vi "audio-stim2.vi"(11 "Stimulus List":dbl[][](array[numeric])) -> (3 "Playing":bool caption="Playing stimulus")   [LabVIEW 2009]
uses:
  <vilib>/DAQmx/create/channels.llb/DAQmx Create Channel (DO-Digital Output).vi
  <vilib>/DAQmx/write.llb/DAQmx Write (Digital U16 1Chan 1Samp).vi
  <vilib>/DAQmx/create/channels.llb/DAQmx Create Channel (AO-Voltage-Basic).vi
  <vilib>/DAQmx/configure/timing.llb/DAQmx Timing (Use Waveform).vi
  <vilib>/DAQmx/write.llb/DAQmx Write (Analog Wfm 1Chan NSamp).vi
panel:
  in  "Total Trials":i32 min=1 step=1
  out "Total Played":i32 caption="Total Played or Cued"
  in  "Save Stimulus List":bool
  in  "Load Stimulus List":bool
  out "Stimulus List Path":path
  out "Log File Path":path
  in  "Play Interval Jitter (s)":dbl
  in  "Play Interval (s)":dbl
  out "error out":errorcluster
  in  "DO Ports":tag caption="DO Ports\n(\"browse\" and select two 8 bit ports)"
  in  "Sound AO Channel":tag
  out "Curr Param":dbl[](array[numeric]) caption="Current (or Cued) Trial Parameters"
  in  "Sampling Rate":dbl
  in  "stop":bool
  in  "Play":bool
  out "Current (or Cued) Waveform":waveform(dbl)(graph)
  out "Waiting":bool
  # "Stim#, Stim Type, Duration, Amplitude, Param 1, Param 2, Param 3, Param 4"
  # "Stim Type 1 DC (no parameters, just amplitude)"
  # "Stim Type 3 Pure Tone (param1 = frequency)"
  # "Stim Type 4 FM Sweep (param1 = start frequency, param2 = end frequency)"
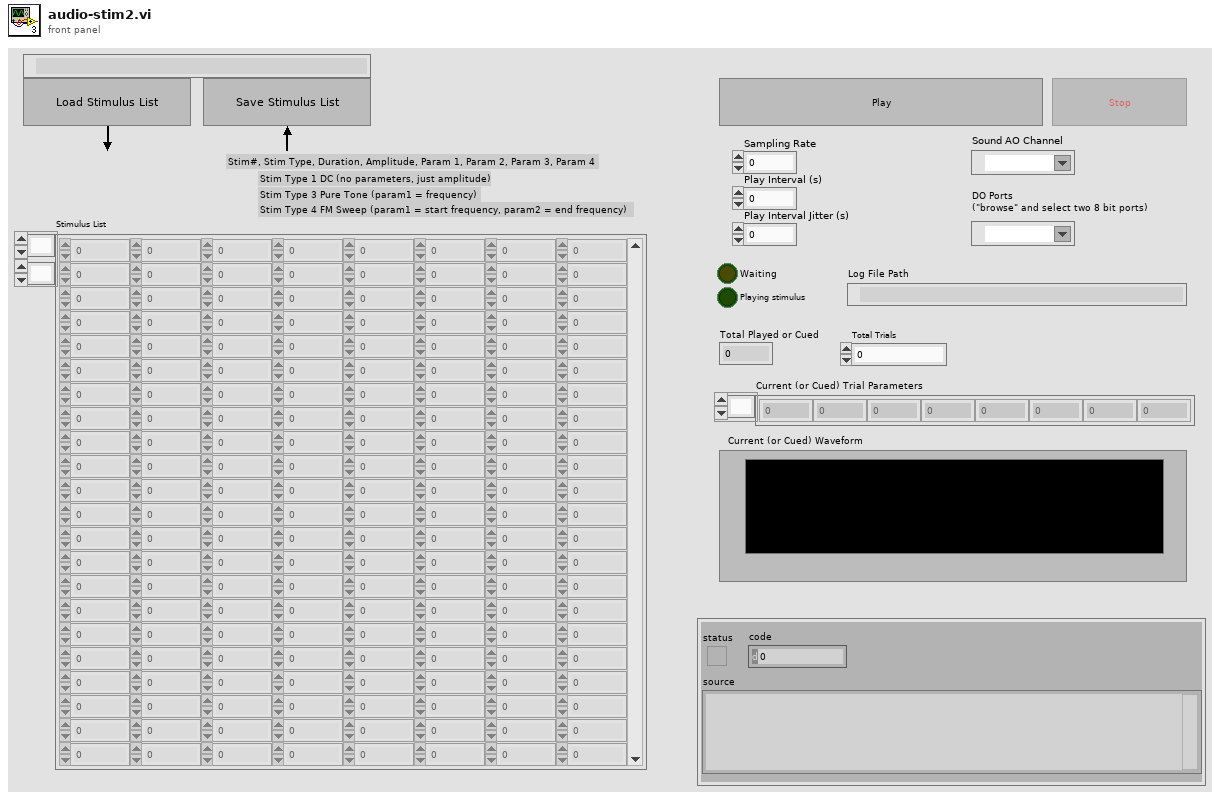
[diagram p1: front panel]
types:
  T1 = enum8{"Enabled", "Disabled", "Disabled and Grayed Out"}
  T2 = cluster{"Sampling Rate":dbl, "Value 3":dbl, dbl, "Value 2":dbl}
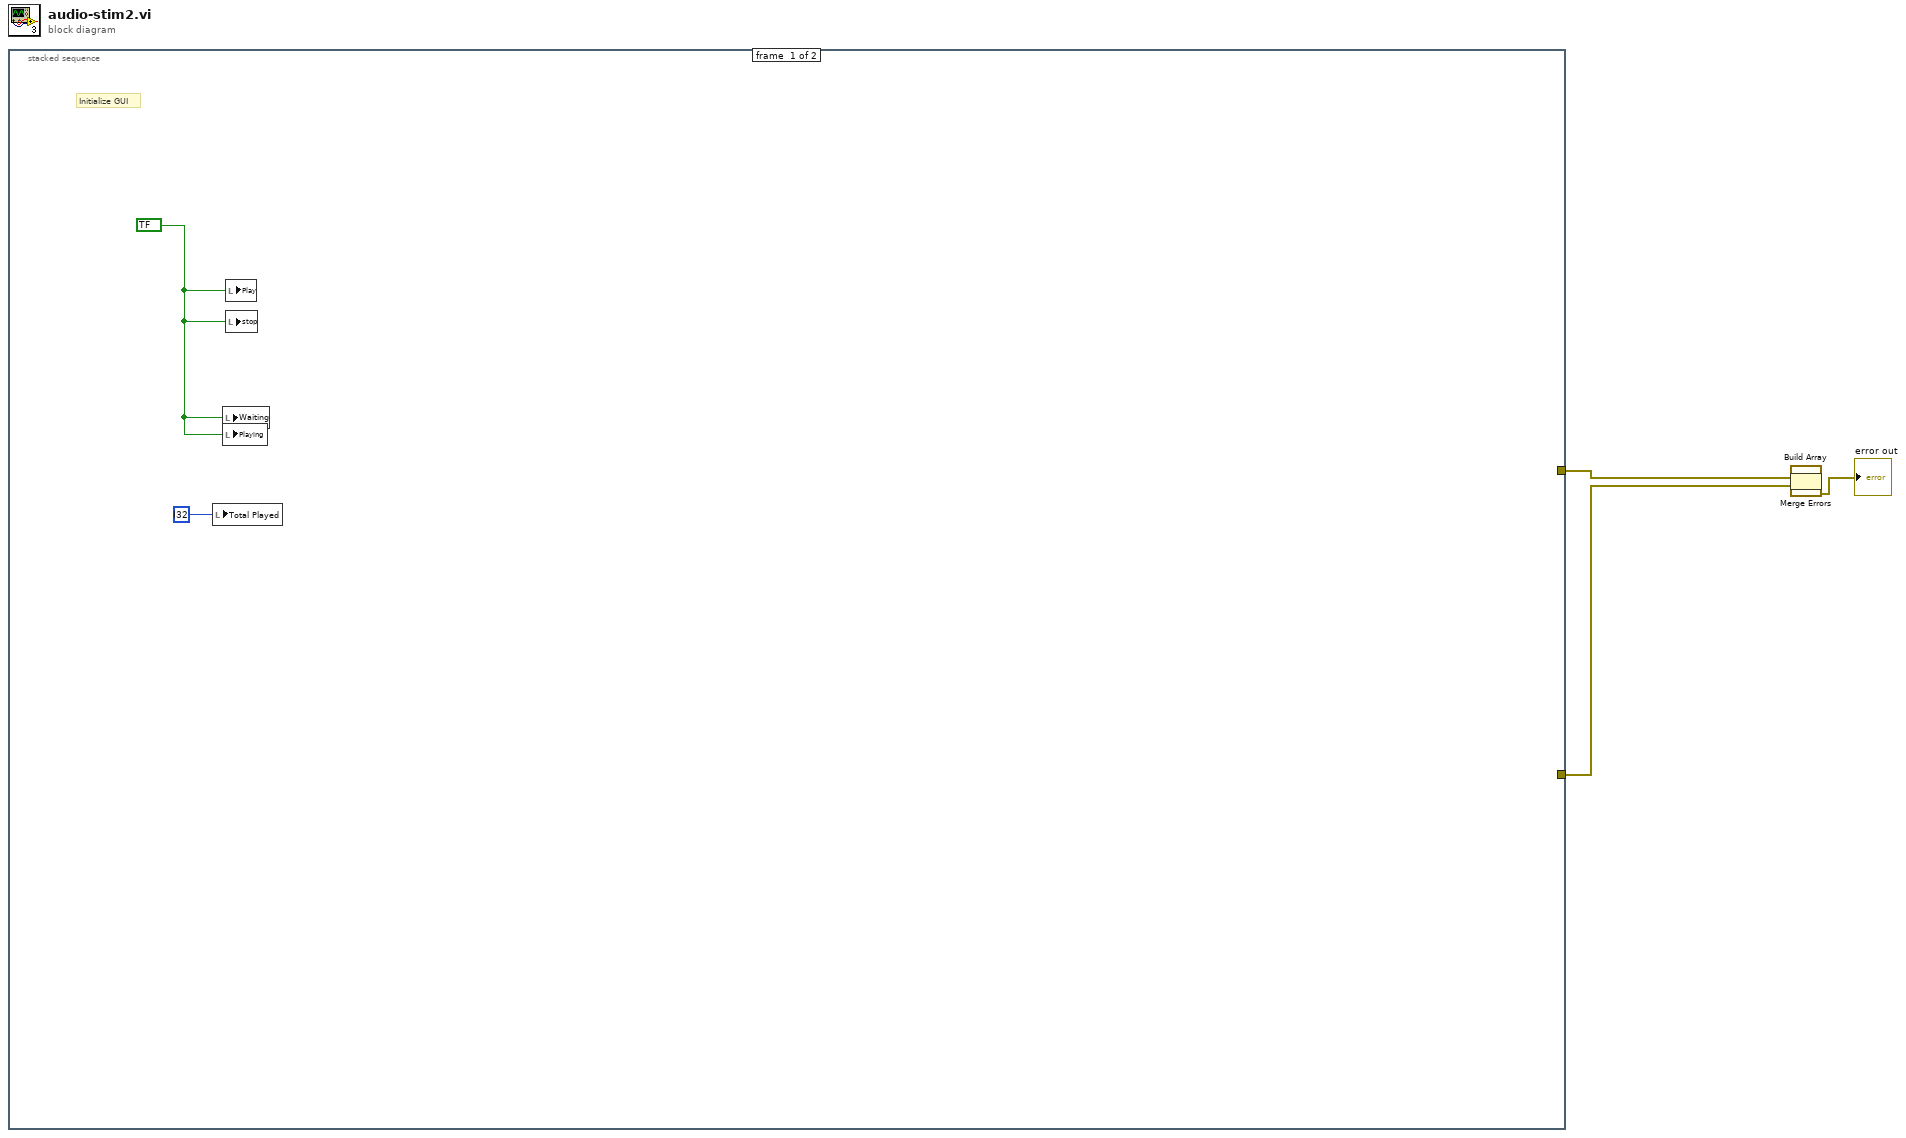
[diagram p0: block diagram]
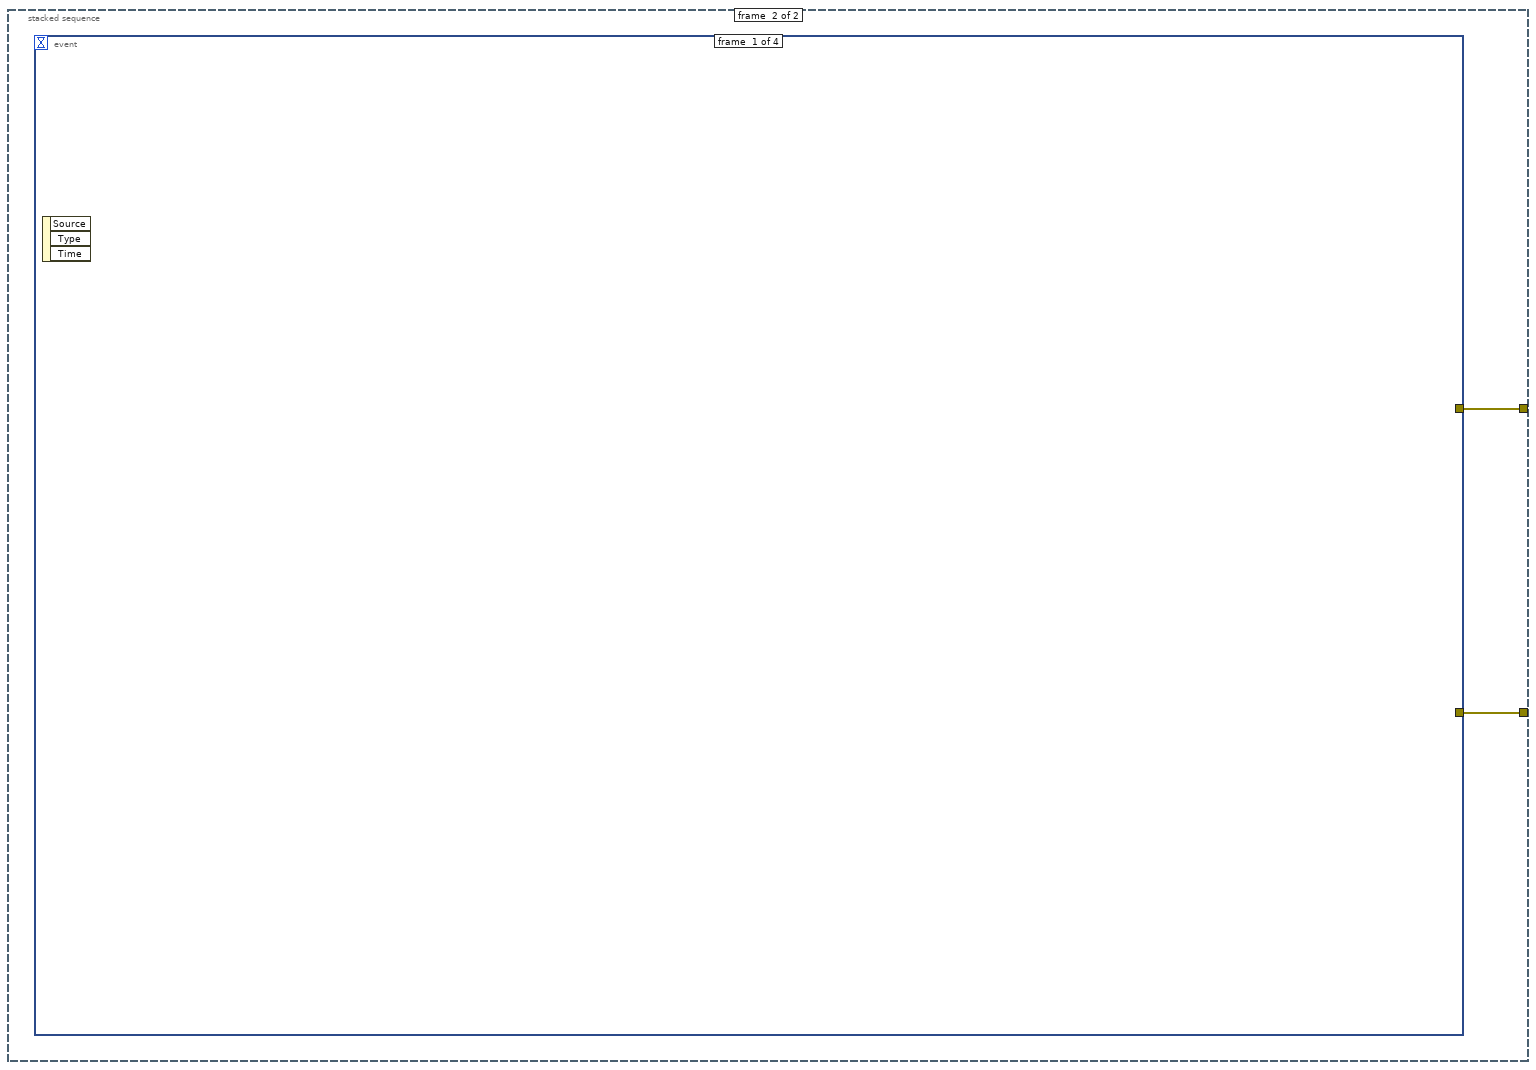
[diagram p2: hidden frame]
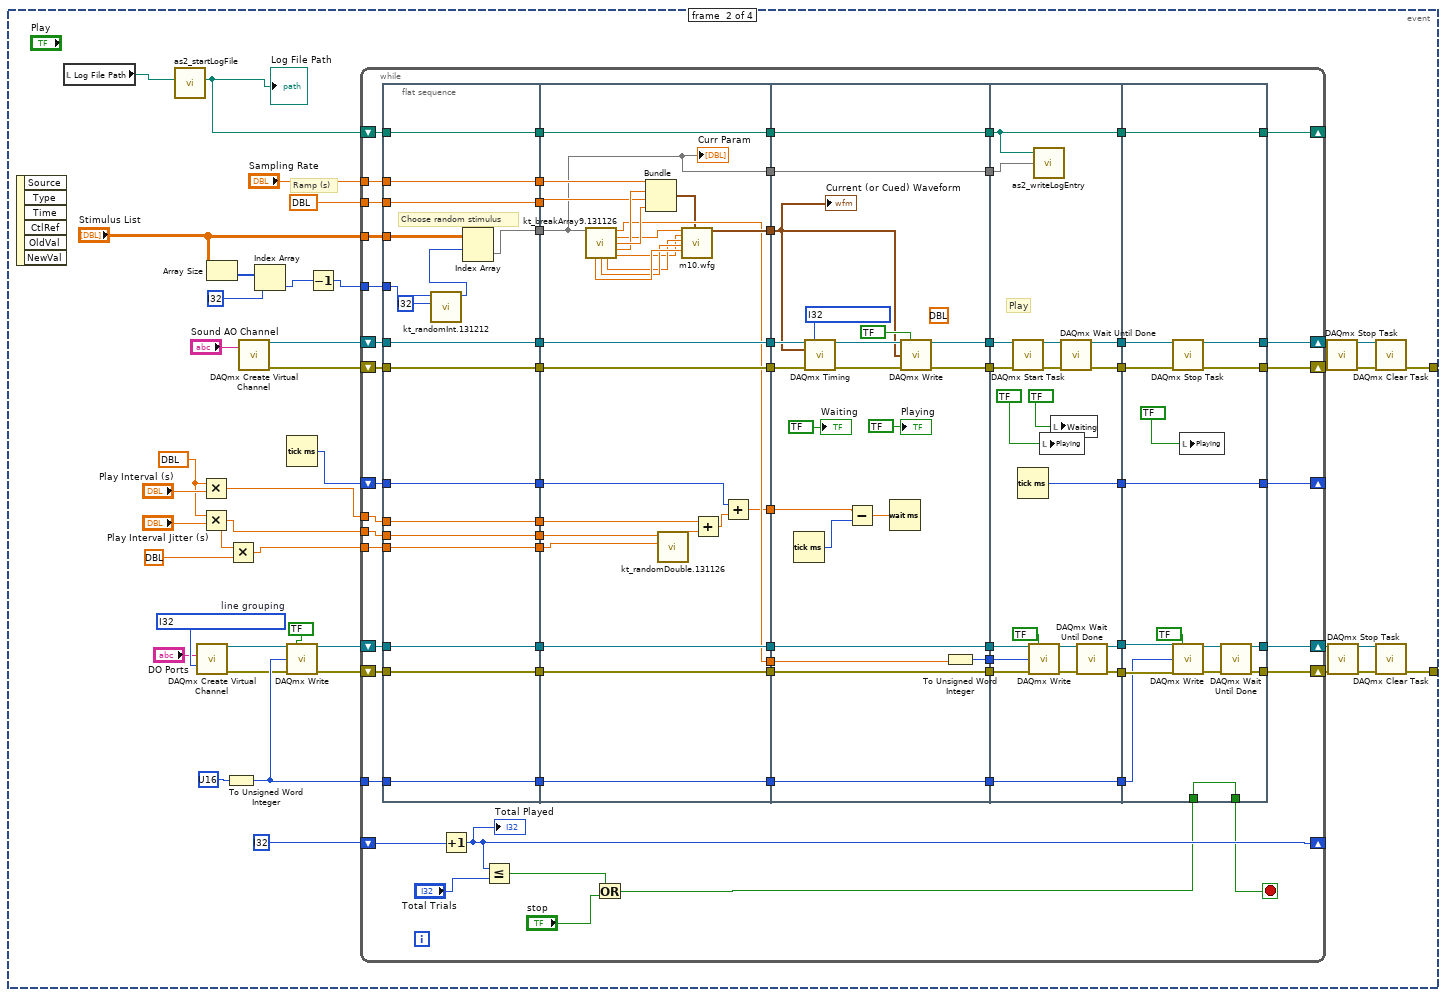
[diagram p3: hidden frame]
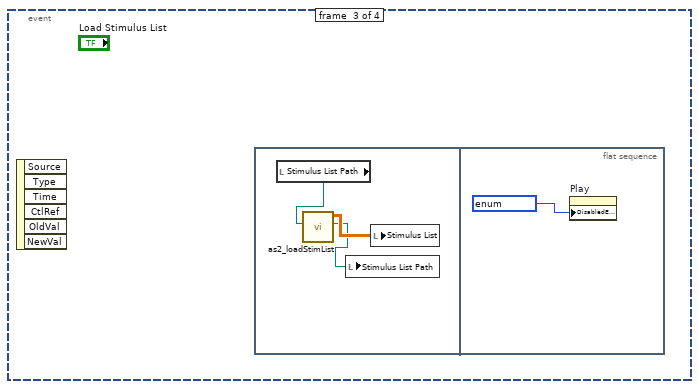
[diagram p4: hidden frame]
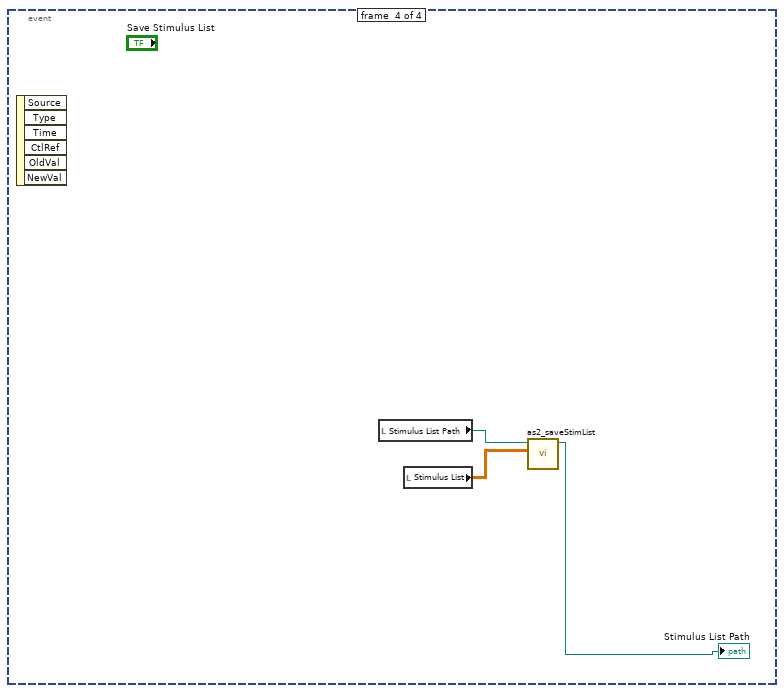
[diagram p5: hidden frame]
diagram:
  n1 = stacked-sequence {
    tunnel: [_ w8] -> w4
    tunnel: [_ w7] -> w3
    frame #0 {
      w6 = bool ? ("Play")
      # "Initialize GUI"
      n2 = local write "Total Played"(i32 ? ("Total Played")) -> ()
      n3 = local write "Waiting"(w6) -> ()
      n4 = local write "Playing"(w6) -> ()
      n5 = local write "Play"(w6) -> ()
      n6 = local write "stop"(w6) -> ()
    }
    frame #1 {
      n7 = event shown="[3] \"Save Stimulus List\": Value Change" {
        selector: _ -> [_ _ _ _]
        dyn-events: _ -> [_ _ _ _]
        timeout: _ -> [_ _ _ _]
        tunnel: [_ w25 _ _] -> w8
        tunnel: [_ w24 _ _] -> w7
        event #0 {
          n8 = event-data() -> ()  [unwired: 1 in, 3 out]
        }
        event #1 {
          w18 = dbl ? ("y")
          w45 = i32 ? items=["one channel for each line", "one channel for all lines"]  # line grouping
          # "Ramp (s)"
          n9 = event-data() -> ()  [unwired: 1 in, 6 out]
          n10 = local read "Log File Path"() -> (w13:path)
          n11 = call "as2_startLogFile.vi"("Path In"=w13) -> ("Path"=w12:path)  [unwired: 5 in, 1 out]
          "Log File Path" <- w12
          n12 = call-poly <vilib>:"DAQmx Create Virtual Channel.vi"("lines"="DO Ports", "line grouping"=w45) -> ("task out"=w23:refnum<k21>, "error out"=w22:errorcluster)  [unwired: 12 in]
          n13 = Multiply(x=w18, y="Play Interval (s)") -> (x*y=w17:dbl)
          n14 = Multiply(x=w18, y="Play Interval Jitter (s)") -> (x*y=w15:dbl)
          n15 = Array Size(array="Stimulus List") -> (size(s)=w43:i32[])
          n16 = To Unsigned Word Integer(number=u16 ? ("data")) -> (unsigned 16bit integer=w28:u16)
          n17 = Multiply(x=w15, y=dbl ?) -> (x*y=w16:dbl)
          n18 = call-poly <vilib>:"DAQmx Create Virtual Channel.vi"("physical channels"="Sound AO Channel") -> ("task out"=w27:refnum<k21>, "error out"=w26:errorcluster)  [unwired: 13 in]
          n19 = Index Array(array=w43, index=i32 ?) -> (element=w11:i32)
          n20 = Tick Count (ms)() -> (millisecond timer value=w14:u32)
          n21 = call-poly <vilib>:"DAQmx Write.vi"("task/channels in"=w23, "auto start"=bool ?, "data"=w28, "error in"=w22) -> ("task out"=w32:refnum<k21>, "error out"=w31:errorcluster)  [unwired: 9 in, 1 out]
          n22 = Decrement(x=w11) -> (x-1=w10:i32)
          n23 = while {
            tunnel: "Stimulus List" -> [w86]
            tunnel: "Sampling Rate" -> [w85]
            tunnel: dbl ? -> [w84]
            shift-right: [w111] -> w37
            shift-left: w27 -> [w109]
            shift-right: [w110] -> w36
            shift-left: w26 -> [w108]
            shift-right: [w100] -> w41
            shift-left: w32 -> [w107]
            shift-right: [w99] -> w40
            shift-left: w31 -> [w94]
            shift-right: [w52] -> _
            shift-left: i32 ? ("data") -> [w53]
            tunnel: w28 -> [w97]
            shift-right: [w81] -> _
            shift-left: w14 -> [w80]
            tunnel: w17 -> [w76]
            tunnel: w16 -> [w77]
            tunnel: w15 -> [w78]
            shift-right: [w69] -> _
            shift-left: w12 -> [w75]
            tunnel: w10 -> [w55]
            stop <- w50 stop-if-true
            n24 = flat-sequence {
              tunnel: w75 -> [w119]
              tunnel: w76 -> [w120]
              tunnel: w77 -> [w121]
              tunnel: w78 -> [w122]
              tunnel: w80 -> [w123]
              tunnel: w84 -> [w124]
              tunnel: w85 -> [w125]
              tunnel: w86 -> [w116]
              tunnel: w94 -> [w126]
              tunnel: w97 -> [w127]
              tunnel: w107 -> [w128]
              tunnel: w108 -> [w129]
              tunnel: w109 -> [w130]
              tunnel: [w130] -> w68
              tunnel: [w129] -> w67
              tunnel: [w128] -> w66
              tunnel: [w127] -> w65
              tunnel: [w126] -> w64
              tunnel: [w114] -> w63
              tunnel: [w125] -> w62
              tunnel: [w124] -> w61
              tunnel: [w123] -> w60
              tunnel: [w122] -> w59
              tunnel: [w121] -> w58
              tunnel: [w120] -> w57
              tunnel: [w119] -> w56
              tunnel: w55 -> [w118]
              tunnel: [w156] -> w92
              tunnel: [w155] -> w91
              tunnel: [w154] -> w90
              tunnel: [w153] -> w89
              tunnel: [w152] -> w88
              tunnel: [w144] -> w87
              tunnel: [w141] -> w83
              tunnel: [w138] -> w79
              tunnel: [w132] -> w74
              tunnel: [w131] -> w73
              tunnel: w68 -> [w156]
              tunnel: w67 -> [w155]
              tunnel: w66 -> [w154]
              tunnel: w65 -> [w153]
              tunnel: w64 -> [w152]
              tunnel: w63 -> [w131]
              tunnel: w62 -> [w143]
              tunnel: w61 -> [w142]
              tunnel: w60 -> [w139]
              tunnel: w59 -> [w137]
              tunnel: w58 -> [w136]
              tunnel: w57 -> [w133]
              tunnel: w56 -> [w132]
              tunnel: [w167] -> w113
              tunnel: [w166] -> w112
              tunnel: [w176] -> w106
              tunnel: [w175] -> w101
              tunnel: [w174] -> w98
              tunnel: [w164] -> w93
              tunnel: w92 -> [w173]
              tunnel: w91 -> [w172]
              tunnel: w90 -> [w176]
              tunnel: w89 -> [w174]
              tunnel: w88 -> [w164]
              tunnel: w87 -> [w163]
              tunnel: w83 -> [w162]
              tunnel: w79 -> [w159]
              tunnel: w74 -> [w157]
              tunnel: w73 -> [w158]
              tunnel: [w158] -> w72
              tunnel: [w157] -> w71
              tunnel: w113 -> [w187]
              tunnel: w112 -> [w186]
              tunnel: w106 -> [w195]
              tunnel: [w189] -> w105
              tunnel: [w188] -> w104
              tunnel: [w192] -> w103
              tunnel: [w191] -> w102
              tunnel: w101 -> [w196]
              tunnel: w98 -> [w190]
              tunnel: [w190] -> w96
              tunnel: w93 -> [w181]
              tunnel: [w180] -> w82
              tunnel: w72 -> [w179]
              tunnel: w71 -> [w178]
              tunnel: [w178] -> w70
              tunnel: [w201] -> w110
              tunnel: [w202] -> w111
              tunnel: w105 -> [w204]
              tunnel: w104 -> [w203]
              tunnel: w103 -> [w212]
              tunnel: w102 -> [w211]
              tunnel: [w207] -> w100
              tunnel: [w206] -> w99
              tunnel: w96 -> [w205]
              tunnel: w82 -> [w200]
              tunnel: [w200] -> w81
              tunnel: w70 -> [w199]
              tunnel: [w199] -> w69
              tunnel: w51 -> [w198]
              tunnel: [w198] -> w50
              frame #0 {
                # "Choose random stimulus"
                n25 = call "kt_randomInt.131212.vi"("Min"=i32 ?, "Max"=w118) -> ("Random"=w115:i32)  [unwired: 9 in]
                n26 = Index Array(array=w116, index (row)=w115) -> (element=w114:dbl[])  [unwired: 1 in]
              }
              frame #1 {
                n27 = call "kt_breakArray9.131126.vi"("Current (or Cued Trial Parameters)"=w131) -> ("Value 0"=w141:dbl, "Value 1"=w145:dbl, "Value 2"=w147:dbl, "Value 3"=w146:dbl, "Value 7"=w151:dbl, "Value 6"=w150:dbl, "Value 5"=w149:dbl, "Value 4"=w148:dbl)  [unwired: 6 in, 1 out]
                n28 = Bundle("Sampling Rate"=w143, "Value 3"=w146, w142, "Value 2"=w147) -> (w140:T2)  [unwired: 1 in]
                n29 = call "kt_randomDouble.131126.vi"("Min"=w136, "Max"=w137) -> ("Random"=w134:dbl)  [unwired: 9 in]
                n30 = call "m10.wfg.vi"("Stimulus Type"=w145, "Param 0"=w148, "Param 1"=w149, "Param 2"=w150, "Param 3"=w151, "Waveform Properties"=w140) -> ("Waveform Out"=w144:waveform(dbl))  [unwired: 12 in, 1 out]
                n31 = Add(x=w133, y=w134) -> (x+y=w135:dbl)
                n32 = Add(x=w139, y=w135) -> (x+y=w138:dbl)
                "Curr Param" <- w131
              }
              frame #2 {
                (unwired) dbl ? ("timeout")
                w171 = i32 ? items=["Finite Samples", "Continuous Samples", "Hardware Timed Single Point"] ("sample mode")
                n33 = Tick Count (ms)() -> (millisecond timer value=w160:u32)
                n34 = call-poly <vilib>:"DAQmx Timing.vi"("task/channels in"=w173, "sample mode"=w171, "waveform"=w163, "error in"=w172) -> ("task out"=w170:refnum<k21>, "error out"=w169:errorcluster)  [unwired: 10 in]
                n35 = Subtract(x=w159, y=w160) -> (x-y=w161:dbl)
                n36 = Wait (ms)(milliseconds to wait=w161) -> ()  [unwired: 1 out]
                n37 = call-poly <vilib>:"DAQmx Write.vi"("task/channels in"=w170, "auto start"=bool ?, "data"=w163, "error in"=w169) -> ("task out"=w167:refnum<k21>, "error out"=w166:errorcluster)  [unwired: 9 in, 1 out]
                n38 = To Unsigned Word Integer(number=w162) -> (unsigned 16bit integer=w175:u16)
                "Waiting" <- bool ? ("Playing Stimulus")
                "Playing" <- bool ? ("Playing Stimulus")
                "Current (or Cued) Waveform" <- w163
              }
              frame #3 {
                # "Play"
                n39 = call <vilib>:"DAQmx Start Task.vi"("task/channels in"=w187, "error in"=w186) -> ("task out"=w185:refnum<k21>, "error out"=w184:errorcluster)  [unwired: 12 in]
                n40 = Tick Count (ms)() -> (millisecond timer value=w180:u32)
                n41 = call-poly <vilib>:"DAQmx Write.vi"("task/channels in"=w195, "auto start"=bool ?, "data"=w196, "error in"=w181) -> ("task out"=w194:refnum<k21>, "error out"=w193:errorcluster)  [unwired: 9 in, 1 out]
                n42 = call "as2_writeLogEntry.vi"("Path In"=w178, "Curr Param"=w179) -> ()  [unwired: 4 in, 1 out]
                n43 = local write "Playing"(bool ? ("Playing Stimulus")) -> ()
                n44 = local write "Waiting"(bool ? ("Playing Stimulus")) -> ()
                n45 = call <vilib>:"DAQmx Wait Until Done.vi"("task/channels in"=w185, "error in"=w184) -> ("task out"=w189:refnum<k21>, "error out"=w188:errorcluster)  [unwired: 12 in]
                n46 = call <vilib>:"DAQmx Wait Until Done.vi"("task/channels in"=w194, "error in"=w193) -> ("task out"=w192:refnum<k21>, "error out"=w191:errorcluster)  [unwired: 12 in]
              }
              frame #4 {
                n47 = call <vilib>:"DAQmx Stop Task.vi"("task/channels in"=w204, "error in"=w203) -> ("task out"=w202:refnum<k21>, "error out"=w201:errorcluster)  [unwired: 12 in]
                n48 = call-poly <vilib>:"DAQmx Write.vi"("task/channels in"=w212, "auto start"=bool ?, "data"=w205, "error in"=w211) -> ("task out"=w209:refnum<k21>, "error out"=w208:errorcluster)  [unwired: 9 in, 1 out]
                n49 = local write "Playing"(bool ? ("Playing Stimulus")) -> ()
                n50 = call <vilib>:"DAQmx Wait Until Done.vi"("task/channels in"=w209, "error in"=w208) -> ("task out"=w207:refnum<k21>, "error out"=w206:errorcluster)  [unwired: 12 in]
              }
            }
            n51 = Increment(x=w53) -> (x+1=w52:i32)
            "Total Played" <- w52
            n52 = Less Or Equal?(x=w52, y="Total Trials") -> (x <= y?=w95:bool)
            n53 = Or(x=w95, y="stop") -> (x .or. y?=w51:bool)
          }
          n54 = call <vilib>:"DAQmx Stop Task.vi"("task/channels in"=w37, "error in"=w36) -> ("task out"=w35:refnum<k21>, "error out"=w34:errorcluster)  [unwired: 12 in]
          n55 = call <vilib>:"DAQmx Stop Task.vi"("task/channels in"=w41, "error in"=w40) -> ("task out"=w39:refnum<k21>, "error out"=w38:errorcluster)  [unwired: 12 in]
          n56 = call <vilib>:"DAQmx Clear Task.vi"("task in"=w35, "error in"=w34) -> ("error out"=w25:errorcluster)  [unwired: 13 in]
          n57 = call <vilib>:"DAQmx Clear Task.vi"("task in"=w39, "error in"=w38) -> ("error out"=w24:errorcluster)  [unwired: 13 in]
        }
        event #2 {
          n58 = event-data() -> ()  [unwired: 1 in, 6 out]
          n59 = flat-sequence {
            frame #0 {
              n60 = local read "Stimulus List Path"() -> (w216:path)
              n61 = call "as2_loadStimList.vi"("Path In"=w216) -> ("Path"=w214:path, "Stimulus List"=w215:dbl[][])  [unwired: 4 in, 1 out]
              n62 = local write "Stimulus List Path"(w214) -> ()
              n63 = local write "Stimulus List"(w215) -> ()
            }
            frame #1 {
              n64 = property on="Play" class="Bool (strict)"("DisabledEnum"=T1 ? ("Disabled")) -> ()  [unwired: 2 in, 2 out]
            }
          }
        }
        event #3 {
          n65 = event-data() -> ()  [unwired: 1 in, 6 out]
          n66 = local read "Stimulus List Path"() -> (w220:path)
          n67 = local read "Stimulus List"() -> (w219:dbl[][])
          n68 = call "as2_saveStimList.vi"("Stimulus List"=w219, "Path In"=w220) -> ("Path"=→"Stimulus List Path":path)  [unwired: 4 in, 1 out]
        }
      }
    }
  }
  n69 = Build Array(w4, w3) -> (w1:errorcluster[])
  n70 = call <vilib>:"Merge Errors.vi"("error array in"=w1) -> ("error out"=→"error out":errorcluster)  [unwired: 6 in]
